vi "Graph_draw.vi"() -> ()   [LabVIEW 2023]
uses:
  <vilib>/Utility/file.llb/Read Delimited Spreadsheet (string).vi
panel:
  out "Waveform Graph 5":cluster{"y":i32, "x":dbl, cluster{dbl[]}[]}(graph)
  out "Waveform Graph 4":cluster{"y":i32, "x":dbl, dbl[]}[](graph)
  out "Waveform Graph 3":cluster{"y":i32, "x":dbl, dbl[]}(graph)
  out "Waveform Graph 2":cluster{"y":i32, "x":dbl, dbl[][]}(graph)
  out "Waveform Chart":dbl[][](graph)
  out "Waveform Graph":cluster{dbl[]}[](graph)
  out "Waveform Chart 2":dbl[](graph)
  out "XY Graph":cluster{"time":dbl[], "PWM":dbl[]}[](graph)
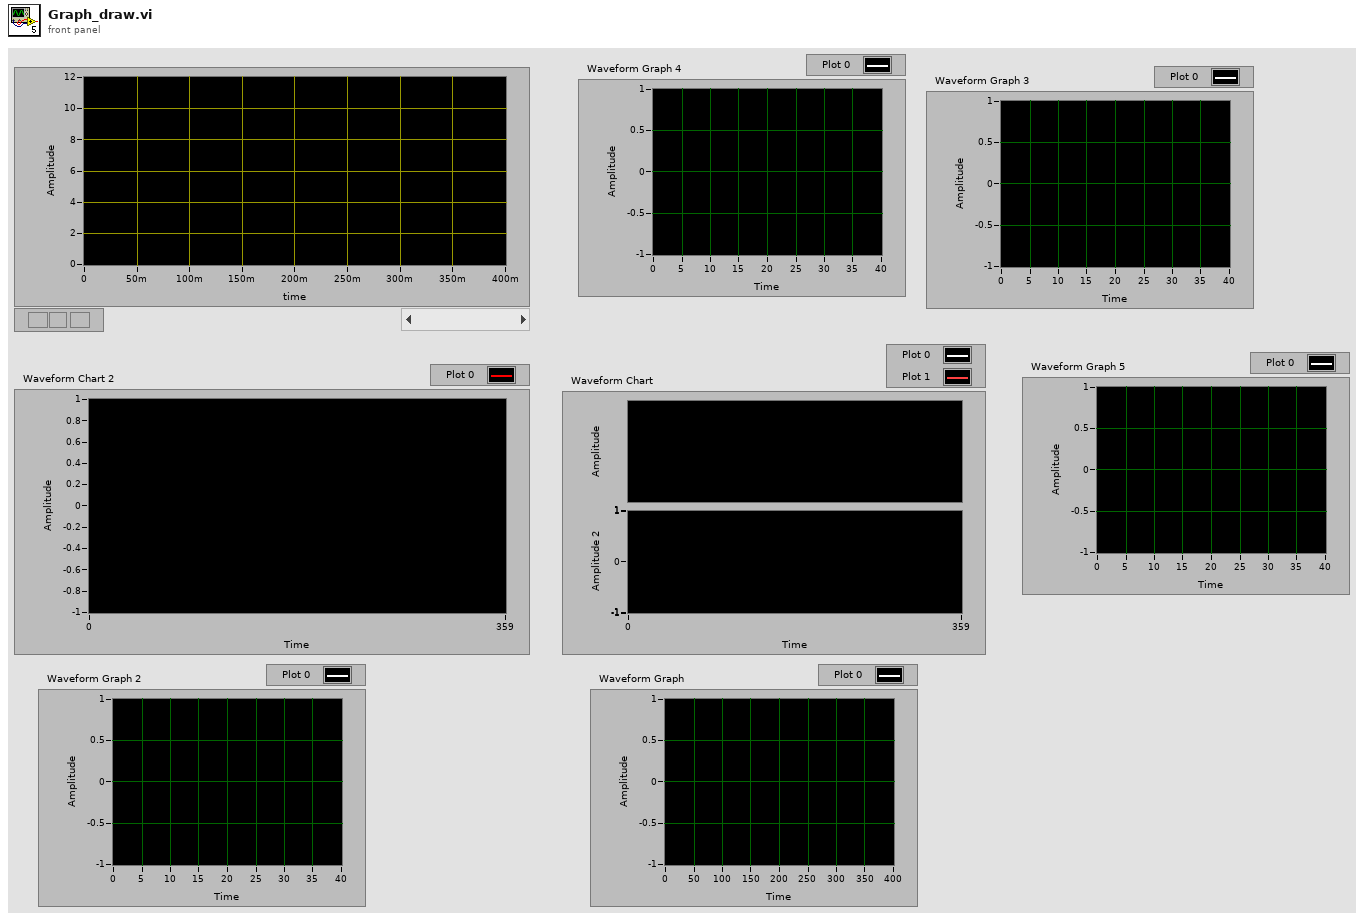
[diagram p1: front panel]
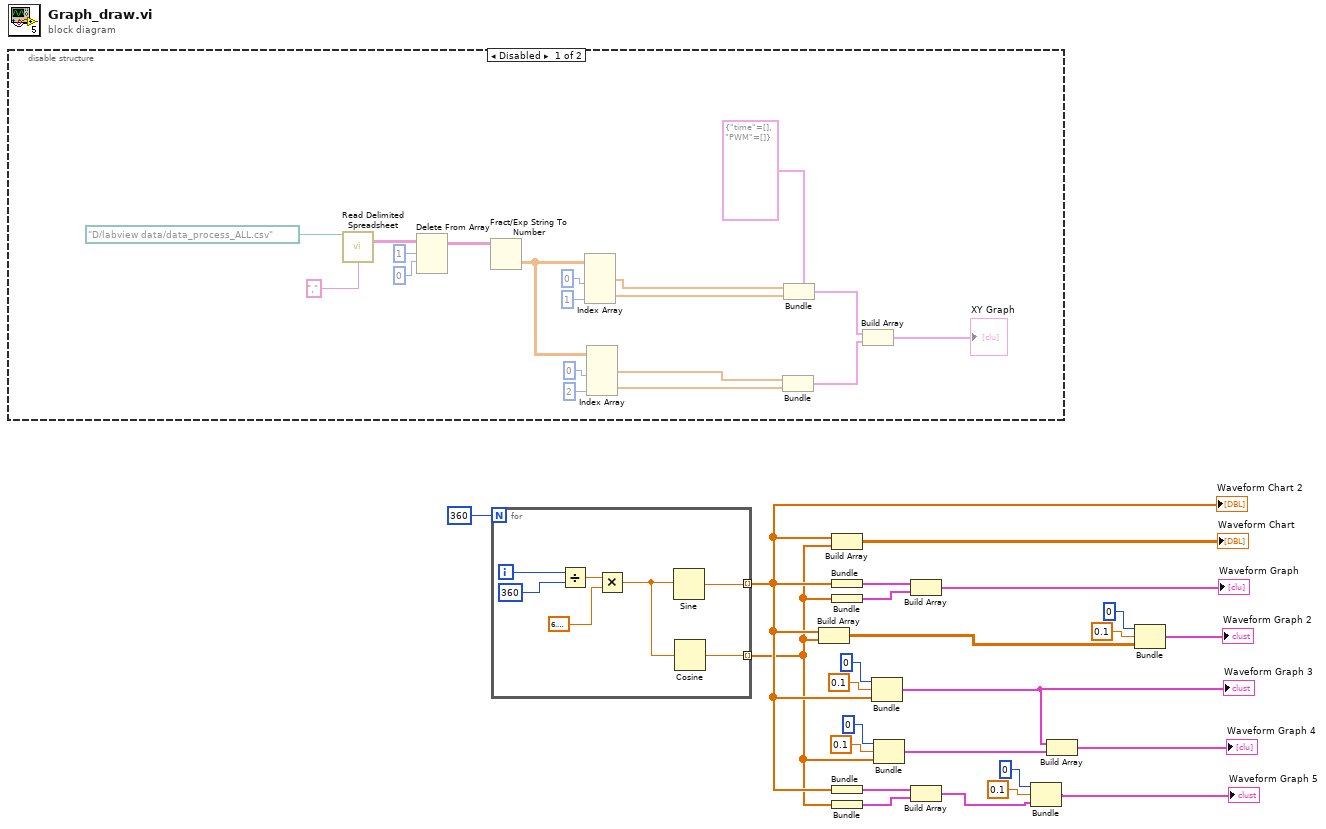
[diagram p0: block diagram]
diagram:
  n1 = disable-structure shown="Disabled" {
    frame Disabled {
      n2 = call-poly <vilib>:"Read Delimited Spreadsheet.vi"("file path (dialog if empty)"=path "D:/labview data/data_process_ALL.csv", "delimiter (\\t)"="," ("delimiter (\\t)")) -> ("all rows"=w41:string[][])  [unwired: 8 in, 5 out]
      n3 = Delete From Array(array=w41, length=1, index (row)=0) -> (array with subset deleted=w35:string[][])  [unwired: 1 in, 1 out]
      n4 = Fract/Exp String To Number(string=w35) -> (number=w32:dbl[][])  [unwired: 3 in, 1 out]
      n5 = Index Array "Index Array"(array=w32, index (col) #1=0 ("disabled index (col)"), index (col) #2=1 ("index (col)")) -> (element #1=w27:dbl[], element #2=w36:dbl[])  [unwired: 2 in]
      n6 = Index Array "Index Array"(array=w32, index (col) #1=0 ("disabled index (col)"), index (col) #2=2 ("index (col)")) -> (element #1=w31:dbl[], element #2=w30:dbl[])  [unwired: 2 in]
      n7 = Bundle(w31, w30) -> (w28:cluster{dbl[], dbl[]})  [unwired: 1 in]
      n8 = Bundle(cluster=cluster{"time":dbl[], "PWM":dbl[]} {"time"=[], "PWM"=[]}, "time"=w27, "PWM"=w36) -> (w29:cluster{"time":dbl[], "PWM":dbl[]})
      n9 = Build Array "Build Array"(w29, w28) -> (→"XY Graph":cluster{"time":dbl[], "PWM":dbl[]}[])
    }
    frame Enabled {
    }
  }
  n10 = for {
    N: 360 -> [_]
    tunnel: [w45] -> w7 mode=indexing
    tunnel: [w44] -> w6 mode=indexing
    i -> [w50]
    n11 = Divide(x=w50, y=360) -> (x/y=w48:dbl)
    n12 = Multiply(x=w48, y=6.283185307179586) -> (x*y=w46:dbl)
    n13 = Sine(x=w46) -> (sin(x)=w45:dbl)
    n14 = Cosine(x=w46) -> (cos(x)=w44:dbl)
  }
  "Waveform Chart 2" <- w7
  n15 = Build Array(w7, w6) -> (w20:dbl[][])
  n16 = Build Array(w7, w6) -> (→"Waveform Chart":dbl[][])
  n17 = Bundle "Bundle"(w7) -> (w23:cluster{dbl[]})  [unwired: 1 in]
  n18 = Bundle(w6) -> (w22:cluster{dbl[]})  [unwired: 1 in]
  n19 = Bundle "Bundle"(w7) -> (w9:cluster{dbl[]})  [unwired: 1 in]
  n20 = Bundle(w6) -> (w8:cluster{dbl[]})  [unwired: 1 in]
  n21 = Bundle("y"=0, "x"=0.1, w7) -> (w11:cluster{"y":i32, "x":dbl, dbl[]})  [unwired: 1 in]
  "Waveform Graph 3" <- w11
  n22 = Bundle("y"=0, "x"=0.1, w6) -> (w12:cluster{"y":i32, "x":dbl, dbl[]})  [unwired: 1 in]
  n23 = Build Array(w23, w22) -> (→"Waveform Graph":cluster{dbl[]}[])
  n24 = Build Array(w9, w8) -> (w3:cluster{dbl[]}[])
  n25 = Bundle("y"=0, "x"=0.1, w3) -> (→"Waveform Graph 5":cluster{"y":i32, "x":dbl, cluster{dbl[]}[]})  [unwired: 1 in]
  n26 = Build Array(w11, w12) -> (→"Waveform Graph 4":cluster{"y":i32, "x":dbl, dbl[]}[])
  n27 = Bundle("y"=0, "x"=0.1, w20) -> (→"Waveform Graph 2":cluster{"y":i32, "x":dbl, dbl[][]})  [unwired: 1 in]
